vi "getEventILCCommunication.vi"(11 "Publisher in":refnum<class "Publisher.lvclass">) -> (2 "EventILCCommunication":T1, 3 "Publisher out":refnum<class "Publisher.lvclass">)   [LabVIEW 2016]
uses:
  Publisher.lvclass
  DataTypes/Topics/Parts/Timestamp.ctl
  DataTypes/Topics/M1M3SupportTopics.lvlib
  DataTypes/Topics/EventILCCommunication.ctl
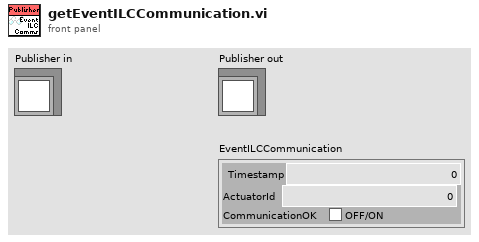
[diagram p1: front panel]
types:
  T1 = typedef "M1M3SupportTopics.lvlib/EventILCCommunication.ctl" = cluster{"Timestamp":T2, "ActuatorId":i32, "CommunicationOK":bool}
  T2 = typedef "M1M3SupportTopics.lvlib/Timestamp.ctl" = dbl
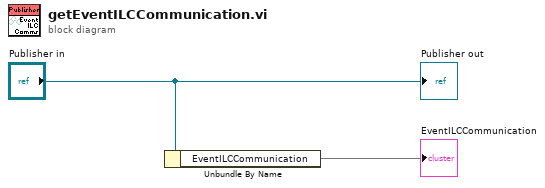
[diagram p0: block diagram]
diagram:
  n1 = Unbundle By Name("Publisher in") -> ("EventILCCommunication"=→"EventILCCommunication")
  "Publisher out" <- "Publisher in"
